vi "Esercitazione 4 - Esercizio per casa, Stringa rettangolo.vi"() -> ()   [LabVIEW 2018]
panel:
  out "String":string
  in  "base":dbl
  in  "altezza":dbl
  # "Restituire un indicatore di stringa contenente un \"rettangolo\" composto da asterichi.\nIl rettangolo deve avere un dato numero di asterischi per riga (BASE).\nIl rettangolo deve avere un dato numero di righe (ALTEZZA)"
  # "sugg = innestare un \nloop in un altro loop"
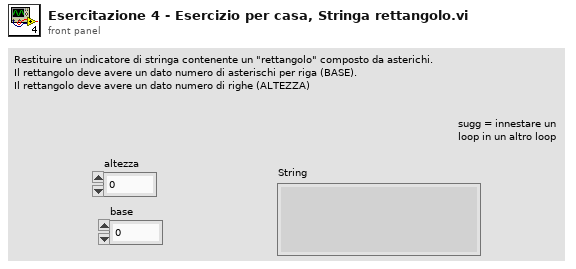
[diagram p1: front panel]
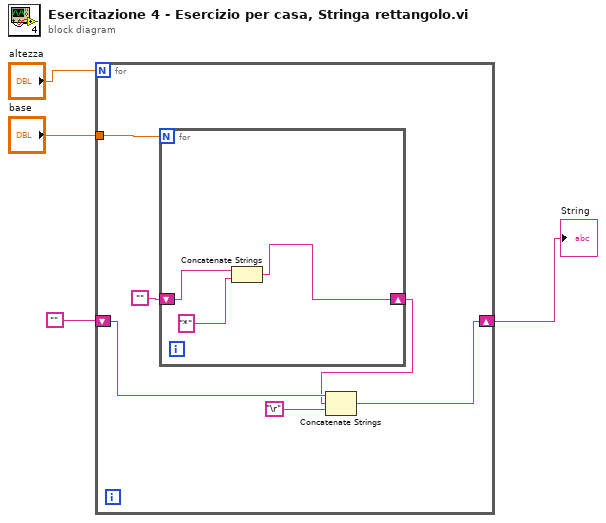
[diagram p0: block diagram]
diagram:
  n1 = for {
    N: "altezza" -> [_]
    tunnel: "base" -> [w10]
    shift-right: [w7] -> w2
    shift-left: "" -> [w8]
    n2 = for {
      N: w10 -> [_]
      shift-right: [w11] -> w5
      shift-left: "" -> [w13]
      n3 = Concatenate Strings(w13, "*") -> (w11:string)
    }
    n4 = Concatenate Strings(w8, w5, "\r") -> (w7:string)
  }
  "String" <- w2
